vi "loopback.vi"() -> ()   [LabVIEW 2013, in "Unix Pipes.lvlib"]
uses:
  Controls/fcntl-linux file modes.ctl
  Unix Pipes.lvlib
panel:
  in  "stop":bool
  out "bytes read":i32
  out "error out":errorcluster
  out "bytes written":i32
  out "data out":string
  out "read fd":i32
  out "write fd":i32
  in  "data in":string="This is a test!"
  in  "pathname in":string="/tmp/fifo"
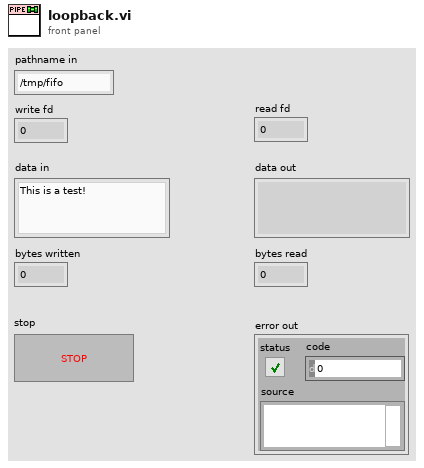
[diagram p1: front panel]
types:
  T1 = typedef "Unix Pipes.lvlib/fcntl-linux file modes.ctl" = u16
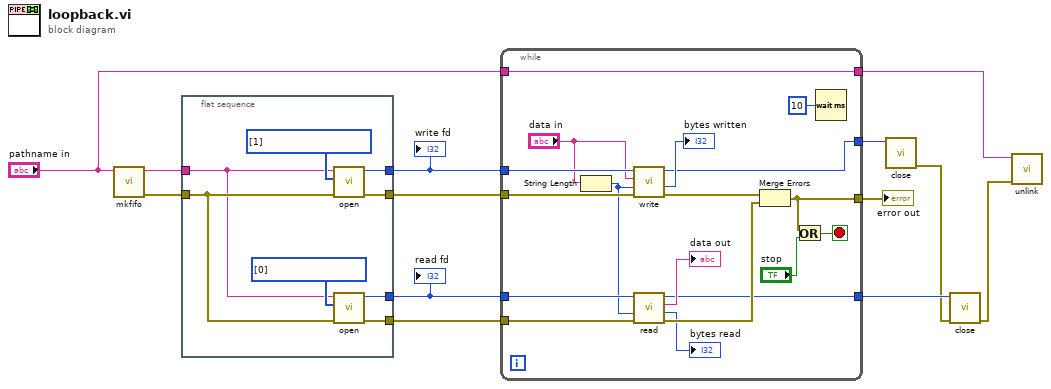
[diagram p0: block diagram]
diagram:
  n1 = call "mkfifo.vi"("pathname in"="pathname in") -> ("error out"=w12:errorcluster, "pathname out"=w13:string)  [unwired: 9 in]
  n2 = flat-sequence {
    tunnel: w13 -> [w18]
    tunnel: w12 -> [w19]
    tunnel: [w17] -> w11
    tunnel: [w16] -> w10
    tunnel: [w15] -> w9
    tunnel: [w14] -> w8
    frame #0 {
      w20 = T1[] [0] items=["O_RDONLY", "O_WRONLY", "O_RDWR"] ("flags")
      w21 = T1[] [1] items=["O_RDONLY", "O_WRONLY", "O_RDWR"] ("flags")
      n3 = call "open.vi"("error in (no error)"=w19, "flags"=w21, "pathname"=w18) -> ("error out"=w16:errorcluster, "file descriptor"=w17:i32)  [unwired: 7 in]
      n4 = call "open.vi"("error in (no error)"=w19, "flags"=w20, "pathname"=w18) -> ("error out"=w14:errorcluster, "file descriptor"=w15:i32)  [unwired: 7 in]
    }
  }
  n5 = while {
    tunnel: w11 -> [w39]
    tunnel: w10 -> [w38]
    tunnel: w9 -> [w36]
    tunnel: w8 -> [w35]
    tunnel: [w26] -> w7
    tunnel: [w27] -> w6
    tunnel: [w23] -> w5
    tunnel: "pathname in" -> [w22]
    tunnel: [w22] -> w3
    stop <- w24 stop-if-true
    n6 = String Length(string="data in") -> (length=w34:i32)
    n7 = call "write.vi"("error in (no error)"=w38, "bytes to write"=w34, "data"="data in", "file descriptor in"=w39) -> ("error out"=w31:errorcluster, "bytes written"=→"bytes written":i32, "file descriptor out"=w27:i32)  [unwired: 5 in]
    n8 = call "read.vi"("error in (no error)"=w35, "bytes to read"=w34, "file descriptor in"=w36) -> ("error out"=w30:errorcluster, "bytes read"=→"bytes read":i32, "data"=→"data out":string, "file descriptor out"=w23:i32)  [unwired: 5 in]
    n9 = Merge Errors(w31, w30) -> (w26:errorcluster)
    n10 = Or(x=w26, y="stop") -> (x .or. y?=w24:bool)
    n11 = Wait (ms)(milliseconds to wait=u32 10) -> ()  [unwired: 1 out]
  }
  "error out" <- w7
  n12 = call "close.vi"("file descriptor in"=w6) -> ("error out"=w2:errorcluster)  [unwired: 10 in]
  n13 = call "close.vi"("error in (no error)"=w2, "file descriptor in"=w5) -> ("error out"=w1:errorcluster)  [unwired: 9 in]
  n14 = call "unlink.vi"("error in (no error)"=w1, "pathname"=w3) -> ()  [unwired: 9 in, 1 out]
  "write fd" <- w11
  "read fd" <- w9
